vi "2D Sweep using GenSweeper.vi"() -> ()   [LabVIEW 2017]
doc: "<B>Custom 2D sweep</B>\nThis VI performs a 2D sweep using a User output and the Generic Sweeper.\nFor each value of the User output (y axis) it will perform a Generic Sweep (x axis). The recorded data will be saved in a .sxm file.\n\n- Nanonis Programming Interface -"
uses:
  Nanonis Prog Interface.lvlib
  Instance           1 33Saved   2D Sweep using GenSweeper .vi
panel:
  in  "Port number (3364)":u32=3364
  in  "Machine name (empty = local machine)":string
  in  "Period (ms)":u16=50
  in  "Y Lower limit":sgl format="%#_6p"
  in  "Y Upper limit":sgl=1.0 format="%#_6p"
  in  "X Lower limit":sgl format="%#_6p"
  in  "X Upper limit":sgl=1.0 format="%#_6p"
  in  "User Output for Y sweep":u8(ring)=2 items=["1", "2", "3", "4", "5", "6", "7", "8"]
  in  "Number of Points Y":i32=100
  in  "Number of Points X":u16=100
  out "Progress":dbl(slide) scale=0.0..1.0
  out "Y Output value":sgl format="%#_6p"
  out "Current sweep data":cluster{"Data":sgl[], "Data":sgl[]}(graph)
  out "Recorded Signal Data":sgl[][](array[numeric])
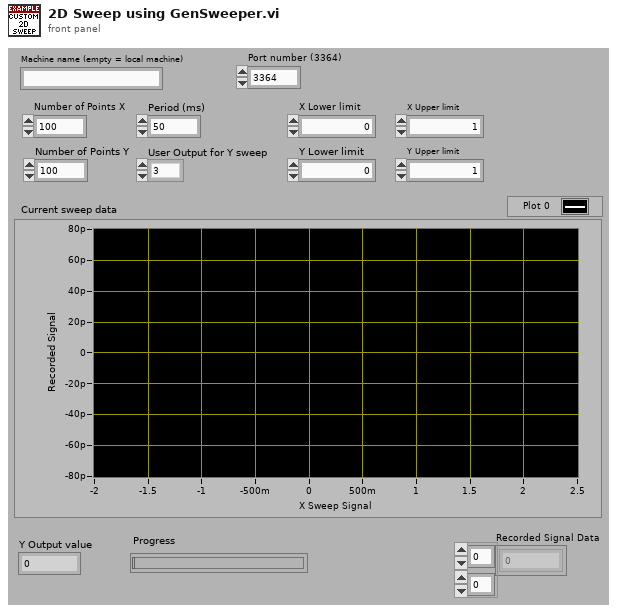
[diagram p1: front panel]
types:
  T1 = cluster{"Initial Settling time (ms) (NaN=no change)":sgl, "Settling time (ms) (NaN=no change)":sgl, "Period (ms) (0=no change)":u16}
  T2 = cluster{"Name":string, "Calibration":sgl, "Offset":sgl, "Channel index":i32}
  T3 = cluster{"center X":sgl, "center Y":sgl, "angle":sgl, "width":sgl, "height":sgl, "# pixels":i32, "# lines":i32}
  T4 = cluster{"up=T/down=F":bool, "time/line":sgl, "start time":timestamp, "end time":timestamp}
  T5 = cluster{"Name":string, "Calibration":sgl, "Offset":sgl, "Channel index":i32}[]
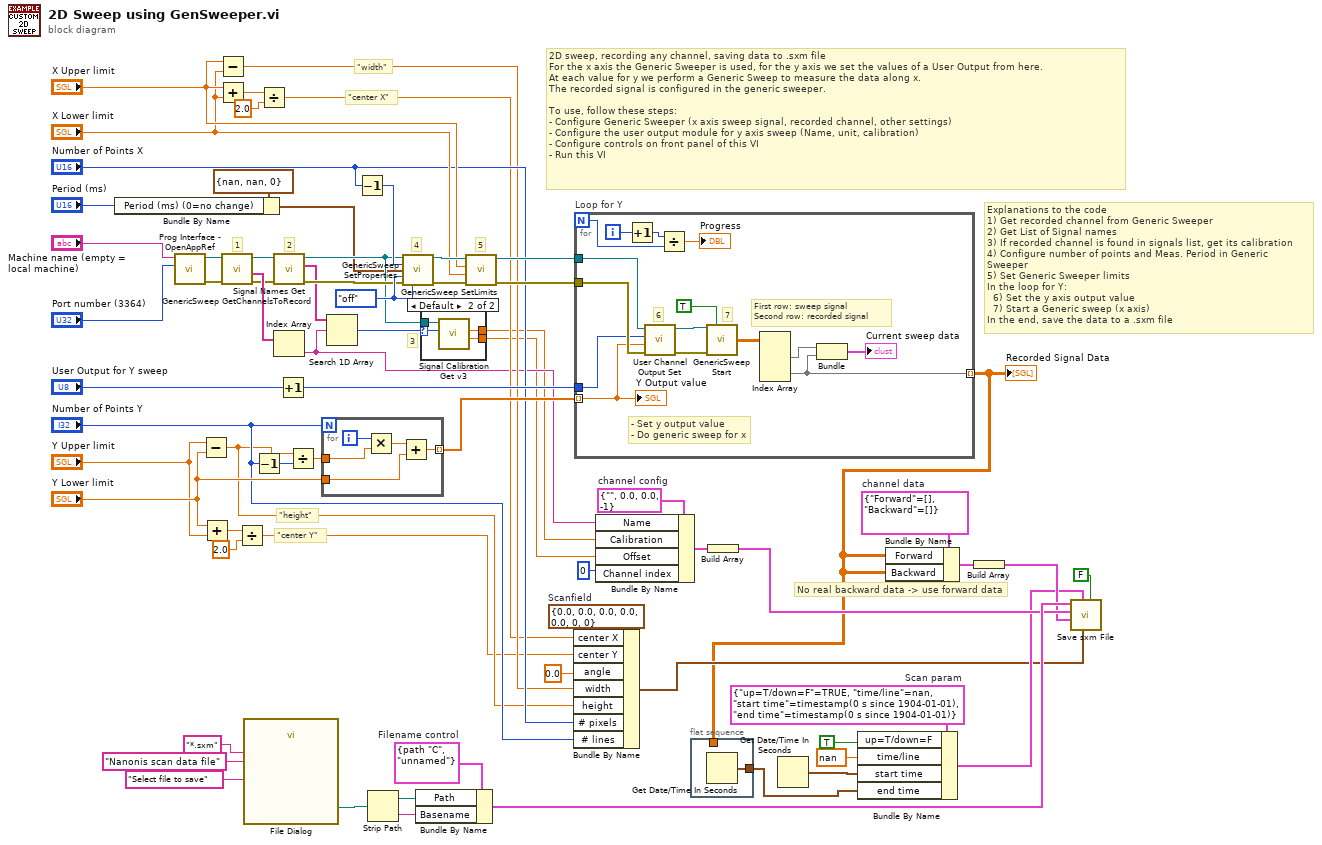
[diagram p0: block diagram]
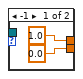
[diagram p2: hidden frame]
diagram:
  w12 = cluster{"Path":path, "Basename":string} {"Path"=path "C:/", "Basename"="unnamed"}  # Filename control
  w26 = cluster{"Forward":sgl[][], "Backward":sgl[][]} {"Forward"=[], "Backward"=[]}  # channel data
  w29 = T2 {"Name"="", "Calibration"=0.0, "Offset"=0.0, "Channel index"=-1}  # channel config
  w9 = T3 {"center X"=0.0, "center Y"=0.0, "angle"=0.0, "width"=0.0, "height"=0.0, "# pixels"=0, "# lines"=0}  # Scanfield
  w38 = T4 {"up=T/down=F"=TRUE, "time/line"=nan, "start time"=timestamp(0 s since 1904-01-01), "end time"=timestamp(0 s since 1904-01-01)}  # Scan param
  w68 = enum16{"no change", "on", "off"}."off" ("Show save dialog (no change)")
  # "Explanations to the code\n1) Get recorded channel from Generic Sweeper\n2) Get List of Signal names\n3) If recorded channel is found in signals list, get its calibration\n4) Configure number of points and Meas. Period in Generic Sweeper\n5) Set Generic Sweeper limits\nIn the loop for Y:\n  6) Set the y axis output value\n  7) Start a Generic sweep (x axis)\nIn the end, save the data to a .sxm file"
  # "3"
  # "5"
  # "4"
  # "2"
  # "1"
  # "\"center Y\""
  # "\"center X\""
  # "\"height\""
  # "\"width\""
  # "No real backward data -> use forward data"
  # "2D sweep, recording any channel, saving data to .sxm file\nFor the x axis the Generic Sweeper is used, for the y axis we set the values of a User Output from here.\nAt each value for y we perform a Generic Sweep to measure the data along x.\nThe recorded signal is configured in the generic sweeper.\n\nTo use, follow these steps:\n- Configure Generic Sweeper (x axis sweep signal, recorded channel, other settings)\n- Configure the user output module for y axis sweep (Name, unit, calibration)\n- Configure controls on front panel of this VI\n- Run this VI"
  n1 = Bundle By Name(cluster=T1 {"Initial Settling time (ms) (NaN=no change)"=nan, "Settling time (ms) (NaN=no change)"=nan, "Period (ms) (0=no change)"=0} ("Times (ms)"), "Period (ms) (0=no change)"="Period (ms)") -> (w2:T1)
  n2 = call <userlib>:"Prog Interface - OpenAppRef.vi"("Port number (3364)"="Port number (3364)", "Machine name (local machine IP)"="Machine name (empty = local machine)") -> ("Error out"=w48:errorcluster, "Application reference"=w49:refnum<vi>)  [unwired: 4 in]
  n3 = Subtract(x="Y Upper limit", y="Y Lower limit") -> (x-y=w33:sgl)
  n4 = Add(x="Y Lower limit", y="Y Upper limit") -> (x+y=w52:sgl)
  n5 = Subtract(x="X Upper limit", y="X Lower limit") -> (x-y=w34:sgl)
  n6 = Add(x="X Upper limit", y="X Lower limit") -> (x+y=w55:sgl)
  n7 = call <userlib>:"GenericSweep GetChannelsToRecord.vi"("error in (no error)"=w48, "Application ref in"=w49) -> ("error out"=w46:errorcluster, "Channels To Record Names"=w47:string[], "Application ref out"=w45:refnum<vi>)  [unwired: 6 in, 1 out]
  n8 = Divide(x=w52, y=sgl 2.0) -> (x/y=w31:sgl)
  n9 = call "File Dialog"("prompt"="Select file to save", "pattern (all files)"="*.sxm" ("pattern"), "pattern label"="Nanonis scan data file") -> ("selected path"=w20:path)  [unwired: 9 in, 3 out]
  n10 = Decrement(x="Number of Points Y") -> (x-1=w61:i32)
  n11 = Divide(x=w55, y=sgl 2.0) -> (x/y=w32:sgl)
  n12 = call <userlib>:"Signal Names Get.vi"("error in (no error)"=w46, "Application ref in"=w45) -> ("error out"=w44:errorcluster, "Signals Names"=w43:string[], "Application ref out"=w41:refnum<vi>)  [unwired: 5 in]
  n13 = Index Array(array=w47) -> (element=w27:string)  [unwired: 1 in]
  n14 = Increment(x="User Output for Y sweep") -> (x+1=w58:u8)
  n15 = Divide(x=w33, y=w61) -> (x/y=w62:sgl)
  n16 = for {
    N: "Number of Points Y" -> [_]
    tunnel: w62 -> [w72]
    tunnel: "Y Lower limit" -> [w70]
    tunnel: [w69] -> w60 mode=indexing
    i -> [w73]
    n17 = Multiply(x=w73, y=w72) -> (x*y=w71:sgl)
    n18 = Add(x=w71, y=w70) -> (x+y=w69:sgl)
  }
  n19 = Search 1D Array(1D array=w43, element=w27) -> (index of element=w42:i32)  [unwired: 1 in]
  n20 = Decrement(x="Number of Points X") -> (x-1=w67:u16)
  n21 = Strip Path(path=w20) -> (stripped path=w14:path, name=w13:string)
  n22 = call <userlib>:"GenericSweep SetProperties.vi"("Application ref in"=w41, "Number of steps (0=no change)"=w67, "Times (ms)"=w2, "Autosave (no change)"=w68, "error in (no error)"=w44, "Show save dialog (no change)"=w68) -> ("Application ref out"=w66:refnum<vi>, "error out"=w65:errorcluster)  [unwired: 8 in]
  n23 = Bundle By Name(cluster=w12, "Path"=w14, "Basename"=w13) -> (w11:cluster{"Path":path, "Basename":string})
  n24 = case shown="Default" w42 {
    selector: w42 -> [_ w79]
    tunnel: w41 -> [_ w78]
    tunnel: [sgl 1.0 ("Calibration (per Volt)") w77] -> w16
    tunnel: [sgl 0.0 ("Offset (physical unit)") w76] -> w15
    frame -1 {
    }
    frame Default {
      n25 = call <userlib>:"Signal Calibration Get v3.vi"("Signal index (0-79)"=w79, "Application ref in"=w78) -> ("Offset (physical unit)"=w76:sgl, "Calibration (per Volt)"=w77:sgl)  [unwired: 5 in, 2 out]
    }
  }
  n26 = call <userlib>:"GenericSweep SetLimits.vi"("error in (no error)"=w65, "Lower limit"="X Lower limit", "Upper limit"="X Upper limit", "Application ref in"=w66) -> ("error out"=w63:errorcluster, "Application ref out"=w64:refnum<vi>)  [unwired: 4 in]
  n27 = Bundle By Name(cluster=w9, "center X"=w32, "center Y"=w31, "angle"=sgl 0.0, "width"=w34, "height"=w33, "# pixels"="Number of Points X", "# lines"="Number of Points Y") -> (w6:T3)
  n28 = for "Loop for Y" {
    N -> [w85]
    tunnel: w64 -> [w93]
    tunnel: w63 -> [w92]
    tunnel: [w88] -> w5 mode=indexing
    tunnel: w58 -> [w83]
    tunnel: w60 -> [w82] mode=indexing
    i -> [w94]
    # "7"
    # "6"
    # "- Set y output value\n- Do generic sweep for x"
    # "First row: sweep signal\nSecond row: recorded signal"
    n29 = Increment(x=w94) -> (x+1=w86:i32)
    n30 = call <userlib>:"User Channel Output Set.vi"("error in (no error)"=w92, "Output value (physical unit)"=w82, "User output channel"=w83, "Application ref in"=w93) -> ("error out"=w80:errorcluster, "Application ref out"=w81:refnum<vi>)  [unwired: 5 in]
    n31 = Divide(x=w86, y=w85) -> (x/y=→"Progress":dbl)
    n32 = call <userlib>:"GenericSweep Start.vi"("Application ref in"=w81, "Get data (F)"=TRUE, "error in (no error)"=w80) -> ("Data"=w90:sgl[][])  [unwired: 9 in, 3 out]
    n33 = Index Array(array=w90) -> (element #1=w89:sgl[], element #2=w88:sgl[])  [unwired: 4 in]
    n34 = Bundle("Data"=w89, "Data"=w88) -> (→"Current sweep data":cluster{"Data":sgl[], "Data":sgl[]})  [unwired: 1 in]
    "Y Output value" <- w82
  }
  "Recorded Signal Data" <- w5
  n35 = Bundle By Name(cluster=w29, "Name"=w27, "Calibration"=w16, "Offset"=w15, "Channel index"=0) -> (w24:T2)
  n36 = flat-sequence {
    tunnel: w5 -> [_]
    tunnel: [w95] -> w4
    frame #0 {
      n37 = Get Date/Time In Seconds() -> (seconds since 1Jan1904=w95:timestamp)
    }
  }
  n38 = Build Array(w24) -> (w10:T5)
  n39 = Get Date/Time In Seconds() -> (seconds since 1Jan1904=w19:timestamp)
  n40 = Bundle By Name(cluster=w38, "up=T/down=F"=TRUE, "time/line"=sgl nan, "start time"=w19, "end time"=w4) -> (w7:T4)
  n41 = Bundle By Name(cluster=w26, "Forward"=w5, "Backward"=w5) -> (w25:cluster{"Forward":sgl[][], "Backward":sgl[][]})
  n42 = Build Array(w25) -> (w8:cluster{"Forward":sgl[][], "Backward":sgl[][]}[])
  n43 = call "Save sxm File.vi"("Auto file naming? (T)"=FALSE, "Scanfield"=w6, "Scan param"=w7, "Channels data"=w8, "Channels config"=w10, "Filename control"=w11) -> ()  [unwired: 3 in, 3 out]
